vi "manage comm restablished.vi"(8 "error in (no error)":errorcluster, 11 "Channel in":refnum<class "Channel.lvclass">) -> (0 "error out":errorcluster, 3 "Channel out":refnum<class "Channel.lvclass">)   [LabVIEW 2018, in "Channel.lvclass"]
uses:
  Channel.lvclass
  Channel.lvclass/Channel.ctl
  Header content/Header content.lvclass/Header content.ctl
  Server/Server.lvclass
  Log File/CCS_Log File.lvclass
  Header content/Header content.lvclass
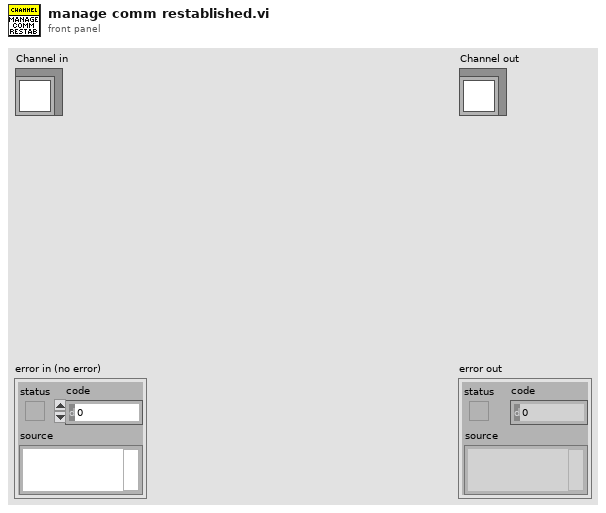
[diagram p1: front panel]
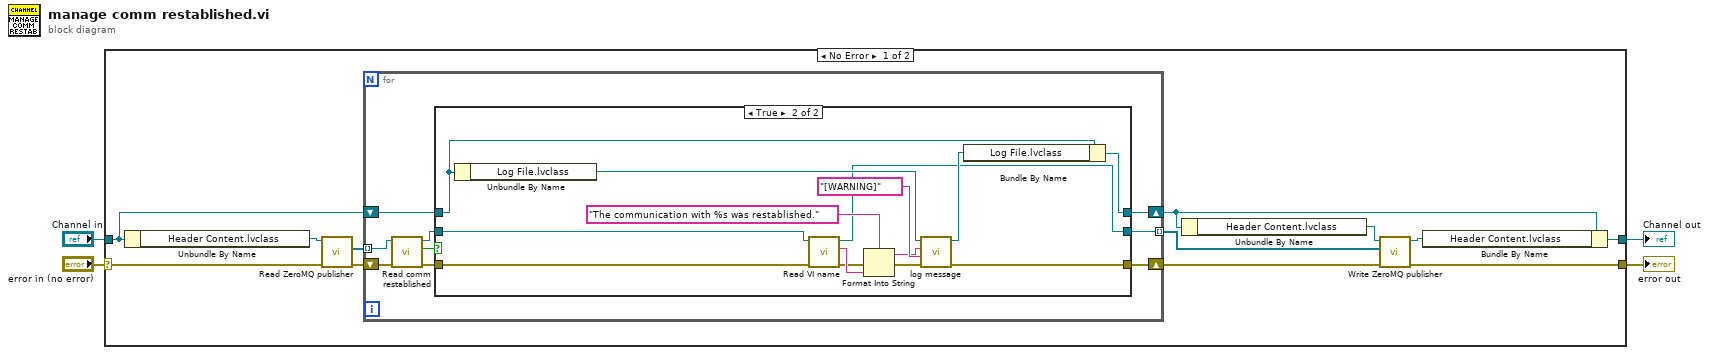
[diagram p0: block diagram]
diagram:
  n1 = case shown="No Error" "error in (no error)" {
    selector: "error in (no error)" -> [w12 w44]
    tunnel: [w6 w44] -> w1
    tunnel: [w5 w43] -> w2
    tunnel: "Channel in" -> [w13 w43]
    frame No Error {
      n2 = Unbundle By Name(w13) -> ("Header Content.lvclass"=w16:refnum<class "Header content.lvclass">)
      n3 = call "Read ZeroMQ publisher.vi"("error in (no error)"=w12, "Header content in"=w16) -> ("error out"=w14:errorcluster, "ZeroMQ publisher"=w15:refnum<class "Server.lvclass">[])  [unwired: 7 in, 1 out]
      n4 = for {
        shift-right: [w24] -> w8
        shift-left: w13 -> [w25]
        shift-right: [w23] -> w11
        shift-left: w14 -> [w21]
        tunnel: w15 -> [w18] mode=indexing
        tunnel: [w22] -> w10 mode=indexing
        n5 = call-dynamic "Read comm restablished.vi"("error in (no error)"=w21, "Server in"=w18) -> ("error out"=w17:errorcluster, "comm restablished"=w20:bool, "Server out"=w19:refnum<class "Server.lvclass">)  [unwired: 7 in]
        n6 = case shown="True" w20 {
          tunnel: w25 -> [w28 w42]
          tunnel: [w28 w41] -> w24
          tunnel: [w27 w40] -> w23
          tunnel: w19 -> [w26 w36]
          tunnel: w17 -> [w27 w35]
          tunnel: [w26 w29] -> w22
          frame False {
          }
          frame True {
            n7 = Unbundle By Name(w42) -> ("Log File.lvclass"=w39:refnum<class "CCS_Log File.lvclass">)
            n8 = call-dynamic "Read VI name.vi"("error in (no error)"=w35, "Server in"=w36) -> ("error out"=w30:errorcluster, "VI name"=w32:string, "Server out"=w29:refnum<class "Server.lvclass">)  [unwired: 7 in]
            n9 = Format Into String(format string="The communication with %s was restablished.", error in=w30, w32) -> (resulting string=w34:string, error out=w33:errorcluster)  [unwired: 1 in]
            n10 = call-dynamic "log message.vi"("error in (no error)"=w33, "message type"="[WARNING]", "Message to log"=w34, "Log File in"=w39) -> ("error out"=w40:errorcluster, "Log File out"=w38:refnum<class "CCS_Log File.lvclass">)  [unwired: 6 in]
            n11 = Bundle By Name(cluster=w42, "Log File.lvclass"=w38) -> (w41:refnum<class "Channel.lvclass">)
          }
        }
      }
      n12 = Unbundle By Name(w8) -> ("Header Content.lvclass"=w9:refnum<class "Header content.lvclass">)
      n13 = call-dynamic "Write ZeroMQ publisher.vi"("error in (no error)"=w11, "ZeroMQ publisher"=w10, "Header content in"=w9) -> ("error out"=w6:errorcluster, "Header content out"=w7:refnum<class "Header content.lvclass">)  [unwired: 7 in]
      n14 = Bundle By Name(cluster=w8, "Header Content.lvclass"=w7) -> (w5:refnum<class "Channel.lvclass">)
    }
    frame Error {
    }
  }
  "error out" <- w1
  "Channel out" <- w2
